vi "oa_Get DSA 449x Oversample Rate and Filter Delay.vi"(9 "EAR enabled? (F)":bool, 11 "vibration signal sample rate":dbl) -> (1 "start":dbl, 3 "oversample rate":dbl format="%#_6f")   [LabVIEW 2017, in "SoundVib_TachProcess.lvlib"]
uses:
  <vilib>/addons/Sound and Vibration/Order Analysis/Tach Process/SoundVib_TachProcess.lvlib
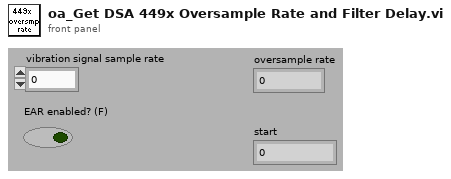
[diagram p1: front panel]
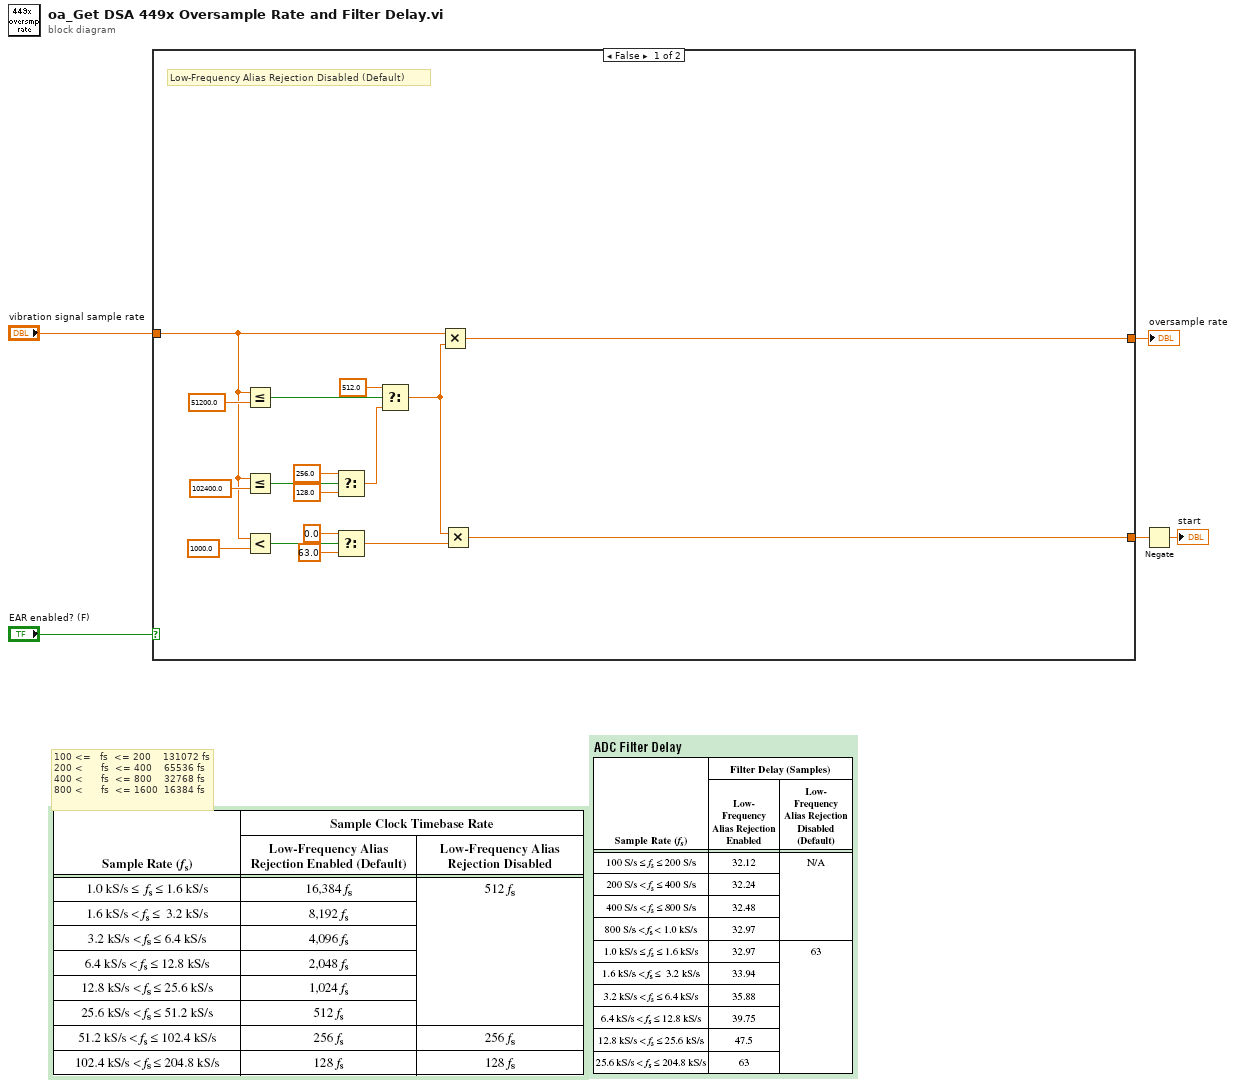
[diagram p0: block diagram]
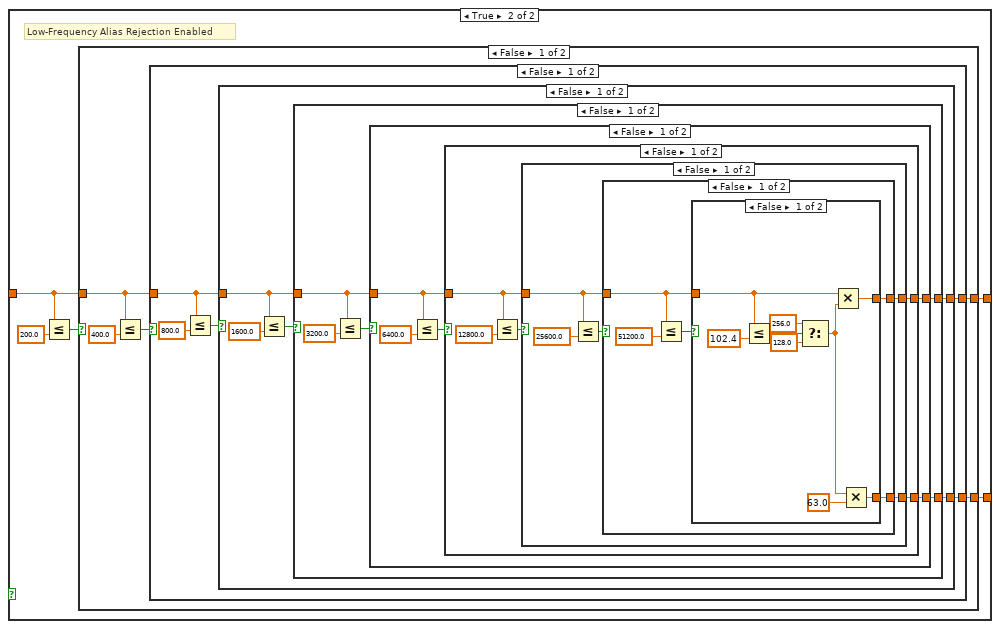
[diagram p2: hidden frame]
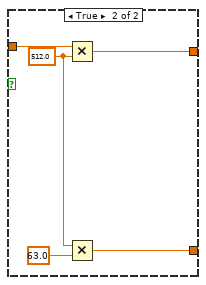
[diagram p3: hidden frame]
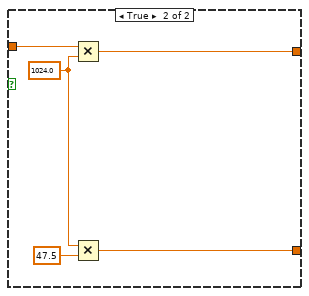
[diagram p4: hidden frame]
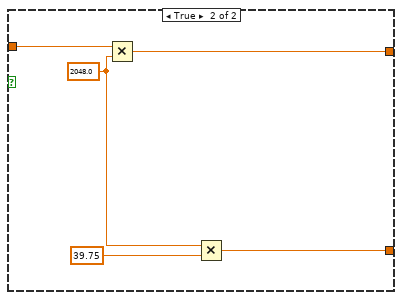
[diagram p5: hidden frame]
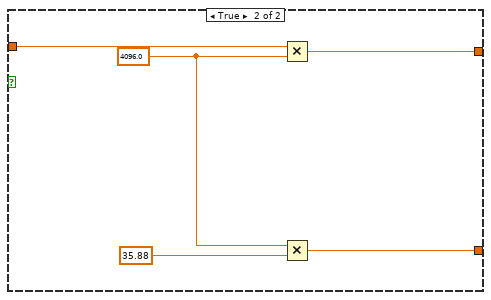
[diagram p6: hidden frame]
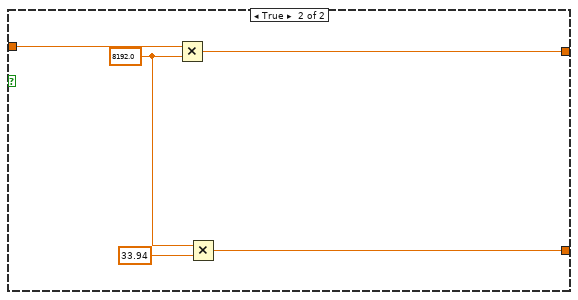
[diagram p7: hidden frame]
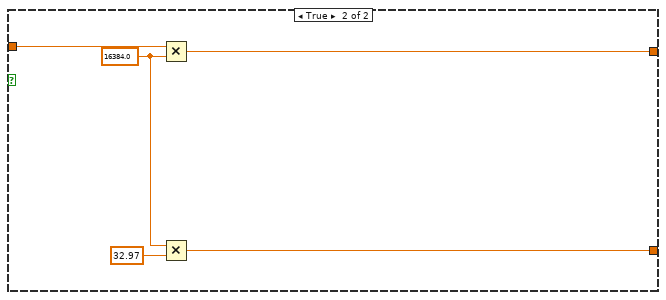
[diagram p8: hidden frame]
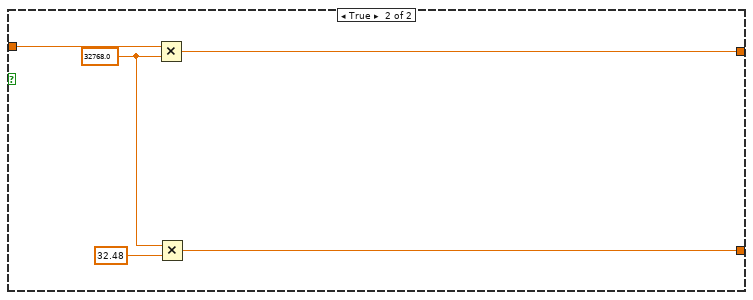
[diagram p9: hidden frame]
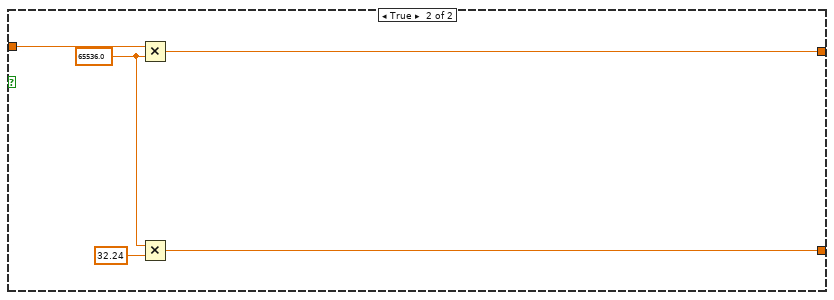
[diagram p10: hidden frame]
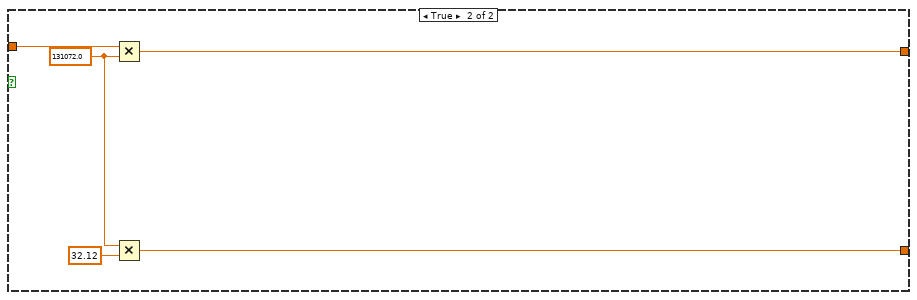
[diagram p11: hidden frame]
diagram:
  # "100 <=   fs  <= 200   \t131072 fs\n200 <      fs  <= 400\t\t  65536 fs\n400 <      fs  <= 800\t\t  32768 fs\n800 <      fs  <= 1600\t\t16384 fs"
  n1 = case shown="False" "EAR enabled? (F)" {
    tunnel: "vibration signal sample rate" -> [w12 w25]
    tunnel: [w19 w23] -> w1
    tunnel: [w18 w24] -> w2
    frame False {
      # "Low-Frequency Alias Rejection Disabled (Default)"
      n2 = Less Or Equal?(x=w12, y=51200.0) -> (x <= y?=w21:bool)
      n3 = Less Or Equal?(x=w12, y=102400.0) -> (x <= y?=w16:bool)
      n4 = Less?(x=w12, y=1000.0) -> (x < y?=w9:bool)
      n5 = Select(t=256.0, s=w16, f=128.0) -> (s? t:f=w10:dbl)
      n6 = Select(t=0.0, s=w9, f=63.0) -> (s? t:f=w6:dbl)
      n7 = Select(t=512.0, s=w21, f=w10) -> (s? t:f=w13:dbl)
      n8 = Multiply(x=w12, y=w13) -> (x*y=w18:dbl)
      n9 = Multiply(x=w13, y=w6) -> (x*y=w19:dbl)
    }
    frame True {
      # "Low-Frequency Alias Rejection Enabled"
      n10 = Less Or Equal?(x=w25, y=200.0) -> (x <= y?=w26:bool)
      n11 = case shown="False" w26 {
        tunnel: w25 -> [w30 w121]
        tunnel: [w29 w120] -> w24
        tunnel: [w28 w117] -> w23
        frame False {
          n12 = Less Or Equal?(x=w30, y=400.0) -> (x <= y?=w31:bool)
          n13 = case shown="False" w31 {
            tunnel: w30 -> [w35 w116]
            tunnel: [w34 w115] -> w29
            tunnel: [w33 w112] -> w28
            frame False {
              n14 = Less Or Equal?(x=w35, y=800.0) -> (x <= y?=w36:bool)
              n15 = case shown="False" w36 {
                tunnel: w35 -> [w40 w111]
                tunnel: [w39 w109] -> w34
                tunnel: [w38 w107] -> w33
                frame False {
                  n16 = Less Or Equal?(x=w40, y=1600.0) -> (x <= y?=w41:bool)
                  n17 = case shown="False" w41 {
                    tunnel: w40 -> [w45 w106]
                    tunnel: [w44 w105] -> w39
                    tunnel: [w43 w102] -> w38
                    frame False {
                      n18 = Less Or Equal?(x=w45, y=3200.0) -> (x <= y?=w46:bool)
                      n19 = case shown="False" w46 {
                        tunnel: w45 -> [w50 w101]
                        tunnel: [w49 w100] -> w44
                        tunnel: [w48 w97] -> w43
                        frame False {
                          n20 = Less Or Equal?(x=w50, y=6400.0) -> (x <= y?=w51:bool)
                          n21 = case shown="False" w51 {
                            tunnel: w50 -> [w55 w96]
                            tunnel: [w54 w95] -> w49
                            tunnel: [w53 w92] -> w48
                            frame False {
                              n22 = Less Or Equal?(x=w55, y=12800.0) -> (x <= y?=w56:bool)
                              n23 = case shown="False" w56 {
                                tunnel: w55 -> [w61 w91]
                                tunnel: [w59 w88] -> w54
                                tunnel: [w58 w87] -> w53
                                frame False {
                                n24 = Less Or Equal?(x=w61, y=25600.0) -> (x <= y?=w60:bool)
                                n25 = case shown="False" w60 {
                                tunnel: w61 -> [w65 w86]
                                tunnel: [w64 w85] -> w59
                                tunnel: [w63 w83] -> w58
                                frame False {
                                n26 = Less Or Equal?(x=w65, y=51200.0) -> (x <= y?=w66:bool)
                                n27 = case shown="False" w66 {
                                tunnel: w65 -> [w71 w81]
                                tunnel: [w72 w80] -> w64
                                tunnel: [w70 w77] -> w63
                                frame False {
                                n28 = Less Or Equal?(x=w71, y=102.4) -> (x <= y?=w75:bool)
                                n29 = Select(t=256.0, s=w75, f=128.0) -> (s? t:f=w69:dbl)
                                n30 = Multiply(x=w71, y=w69) -> (x*y=w72:dbl)
                                n31 = Multiply(x=w69, y=63.0) -> (x*y=w70:dbl)
                                }
                                frame True {
                                w79 = 512.0 ("y")
                                n32 = Multiply(x=w81, y=w79) -> (x*y=w80:dbl)
                                n33 = Multiply(x=w79, y=63.0) -> (x*y=w77:dbl)
                                }
                                }
                                }
                                frame True {
                                w84 = 1024.0 ("y")
                                n34 = Multiply(x=w86, y=w84) -> (x*y=w85:dbl)
                                n35 = Multiply(x=w84, y=47.5) -> (x*y=w83:dbl)
                                }
                                }
                                }
                                frame True {
                                w90 = 2048.0 ("y")
                                n36 = Multiply(x=w91, y=w90) -> (x*y=w88:dbl)
                                n37 = Multiply(x=w90, y=39.75) -> (x*y=w87:dbl)
                                }
                              }
                            }
                            frame True {
                              w94 = 4096.0 ("y")
                              n38 = Multiply(x=w96, y=w94) -> (x*y=w95:dbl)
                              n39 = Multiply(x=w94, y=35.88) -> (x*y=w92:dbl)
                            }
                          }
                        }
                        frame True {
                          w99 = 8192.0 ("y")
                          n40 = Multiply(x=w101, y=w99) -> (x*y=w100:dbl)
                          n41 = Multiply(x=w99, y=33.94) -> (x*y=w97:dbl)
                        }
                      }
                    }
                    frame True {
                      w104 = 16384.0 ("y")
                      n42 = Multiply(x=w106, y=w104) -> (x*y=w105:dbl)
                      n43 = Multiply(x=w104, y=32.97) -> (x*y=w102:dbl)
                    }
                  }
                }
                frame True {
                  w108 = 32768.0 ("y")
                  n44 = Multiply(x=w111, y=w108) -> (x*y=w109:dbl)
                  n45 = Multiply(x=w108, y=32.48) -> (x*y=w107:dbl)
                }
              }
            }
            frame True {
              w114 = 65536.0 ("y")
              n46 = Multiply(x=w116, y=w114) -> (x*y=w115:dbl)
              n47 = Multiply(x=w114, y=32.24) -> (x*y=w112:dbl)
            }
          }
        }
        frame True {
          w119 = 131072.0 ("y")
          n48 = Multiply(x=w121, y=w119) -> (x*y=w120:dbl)
          n49 = Multiply(x=w119, y=32.12) -> (x*y=w117:dbl)
        }
      }
    }
  }
  "oversample rate" <- w2
  n50 = Negate(x=w1) -> (-x=→"start":dbl)
